vi "Get Datatype Bytes.vi"(1 "DataType":T1) -> (0 "N Bytes":u8)   [LabVIEW 2020, in "LV Tiff.lvlib"]
uses:
  LV Tiff.lvlib
  Tiff Data Type.ctl
  Tiff Datatype Bytes.ctl
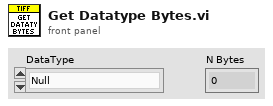
[diagram p1: front panel]
types:
  T1 = typedef "LV Tiff.lvlib/Tiff Data Type.ctl" = enum16{"Null", "BYTE", "ASCII", "SHORT", "LONG", "RATIONAL", "SBYTE", "UNDEFINE", "SSHORT", "SLONG", "SRATIONAL", "FLOAT", "DOUBLE"}
  T2 = typedef "LV Tiff.lvlib/Tiff Datatype Bytes.ctl" = u8[]
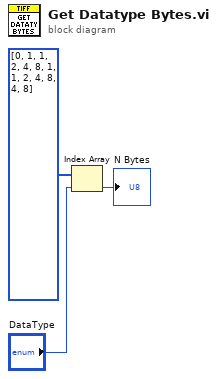
[diagram p0: block diagram]
diagram:
  n1 = Index Array(array=T2 [0, 1, 1, 2, 4, 8, 1, 1, 2, 4, 8, 4, 8] ("Bytes"), index="DataType") -> (element=→"N Bytes":u8)
